vi "GetCameraFeed.vi"() -> ()   [LabVIEW 2017]
uses:
  <vilib>/userdefined/High Color/IMAQdx.ctl
  <vilib>/vision/driver/IMAQdx.llb/IMAQdx Camera Control Mode.ctl
  <vilib>/vision/driver/NI_Vision_Acquisition_Software.lvlib
panel:
  out "Image":T1(plugin-control)
  in  "Session In":T2
  in  "error in":errorcluster
  in  "stop":bool
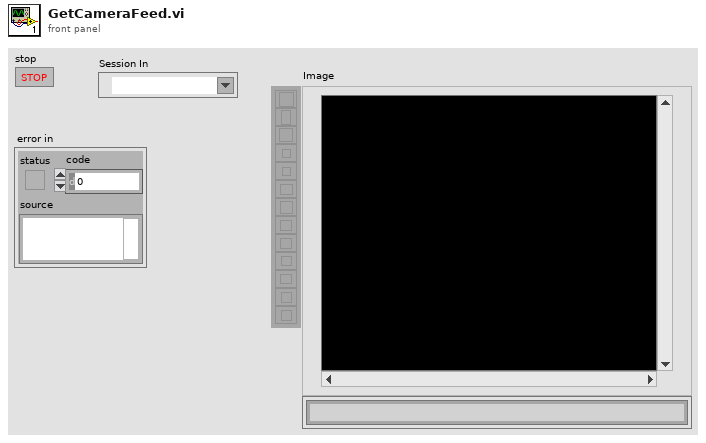
[diagram p1: front panel]
types:
  T1 = typedef "IMAQ Image.ctl" = refnum<image>
  T2 = typedef "IMAQdx.ctl" = refnum<k21>
  T3 = typedef "Image Type" = u32
  T4 = typedef "NI_Vision_Acquisition_Software.lvlib/IMAQdx Camera Control Mode.ctl" = enum32{"Controller", "Listener"}
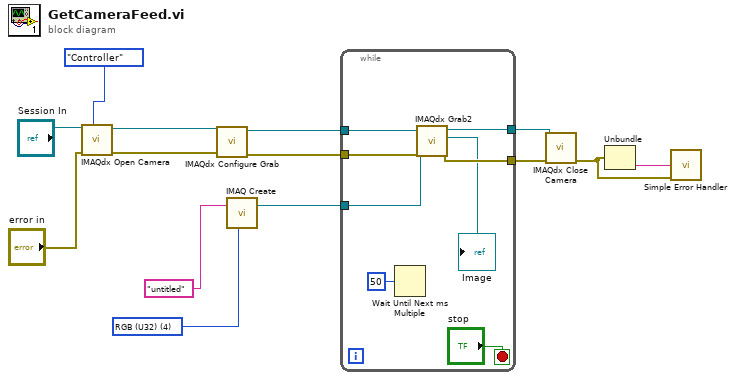
[diagram p0: block diagram]
diagram:
  w5 = T3 4 items=["Grayscale (U8)", "Grayscale (I16)", "Grayscale (SGL)", "Complex (CSG)", "RGB (U32)", "HSL (U32)", "RGB (U64)", "Grayscale (U16)"] ("Image Type")
  n1 = call <vilib>:"IMAQdx Open Camera.vi"("Camera Control Mode"=IMAQdx_Camera_Control_Mode."Controller", "error in"="error in", "Session In"="Session In") -> ("error out"=w10:errorcluster, "Session Out"=w11:T2)  [unwired: 7 in]
  n2 = call <vilib>:"IMAQdx Configure Grab.vi"("error in"=w10, "Session In"=w11) -> ("error out"=w8:errorcluster, "Session Out"=w9:T2)  [unwired: 8 in]
  n3 = call "IMAQ Create"("Image Name"="untitled", "Image Type"=w5) -> ("New Image"=w4:T1)  [unwired: 3 in, 1 out]
  n4 = while {
    tunnel: w9 -> [w21]
    tunnel: w8 -> [w20]
    tunnel: [w19] -> w7
    tunnel: w4 -> [w18]
    tunnel: [w17] -> w3
    stop <- "stop" stop-if-true
    n5 = Wait Until Next ms Multiple(millisecond multiple=u32 50) -> ()  [unwired: 1 out]
    n6 = call <vilib>:"IMAQdx Grab2.vi"("error in"=w20, "Image In"=w18, "Session In"=w21) -> ("error out"=w19:errorcluster, "Image Out"=→"Image":T1, "Session Out"=w17:T2)  [unwired: 5 in, 1 out]
  }
  n7 = call <vilib>:"IMAQdx Close Camera.vi"("error in"=w7, "Session In"=w3) -> ("error out"=w1:errorcluster)  [unwired: 9 in]
  n8 = Unbundle(w1) -> ("source"=w2:string)  [unwired: 2 out]
  n9 = call <vilib>:"Simple Error Handler.vi"("error source (\" \")"=w2, "error in (no error)"=w1) -> ()  [unwired: 3 in, 5 out]
